vi "Choose_Lib.vi"() -> (3 "appended path":path)   [LabVIEW 2016]
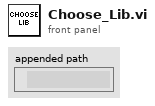
[diagram p1: front panel]
types:
  T1 = enum32{"invalid OS target", "Mac OS", "Windows 3.1", "Windows 95/NT", "Solaris 1", "Solaris 2", "HP-UX", "PowerMAX", "Linux", "Irix", "Rhapsody", "BeOS", "AIX", "OSF1", "VxWorks", "PharLap", "Carbon", "RTX", "Windows x64", "Linux x64", "Mac OS X x64"}
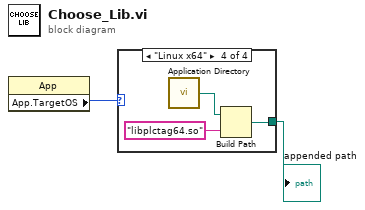
[diagram p0: block diagram]
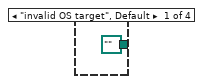
[diagram p2: hidden frame]
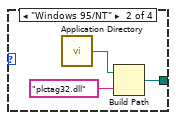
[diagram p3: hidden frame]
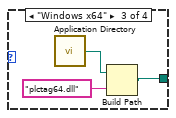
[diagram p4: hidden frame]
diagram:
  n1 = property class="App"() -> ("App.TargetOS"=w1:T1)  [unwired: 2 in, 2 out]
  n2 = case shown="\"Linux x64\"" w1 {
    tunnel: [path "" ("libplc library path") w6 w7 w10] -> w2
    frame "invalid OS target", Default {
    }
    frame "Windows 95/NT" {
      n3 = call <vilib>:"Application Directory.vi"() -> ("Application Directory"=w4:path)
      n4 = Build Path(base path=w4, name or relative path="plctag32.dll" ("libplc library path")) -> (appended path=w6:path)
    }
    frame "Windows x64" {
      n5 = call <vilib>:"Application Directory.vi"() -> ("Application Directory"=w8:path)
      n6 = Build Path(base path=w8, name or relative path="plctag64.dll" ("libplc library path")) -> (appended path=w7:path)
    }
    frame "Linux x64" {
      n7 = call <vilib>:"Application Directory.vi"() -> ("Application Directory"=w11:path)
      n8 = Build Path(base path=w11, name or relative path="libplctag64.so" ("libplc library path")) -> (appended path=w10:path)
    }
  }
  "appended path" <- w2
